vi "Test HDF5.vi"   [LabVIEW 2012]
uses:
  <vilib>/measure/NI_MABase.lvlib
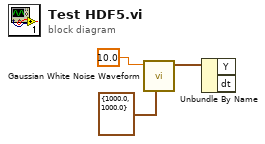
[diagram p0: block diagram]
diagram:
  n1 = call <vilib>:"Gaussian White Noise Waveform.vi"("sampling info"=cluster{"Fs":dbl, "#s":dbl} {"Fs"=1000.0, "#s"=1000.0}, "standard deviation"=10.0) -> ("signal out"=w1:waveform(dbl))  [unwired: 8 in, 1 out]
  n2 = Unbundle By Name(w1) -> ("Y"=w3:dbl[], "dt"=w2:dbl)
